vi "SWITCH Action-Status Calibrate.vi"(8 "error in (no error)":errorcluster, 10 "Message Data":variant, 11 "Data Cluster in":T1={"Tango HW"={"VISA resource"="", "Baud Rate (115200)"=2, "lAnInterfaceType"=0, "bAShowProt"=15}, "Writer Queue"=refnum, "Status"=FALSE, "Abs Position"=[], "Axis Velocity"={"dX"=0.0, "dY"=0.0, "dZ"=0.0, "dA"=0.0}, "acceleration "=0.0, "Z direction"=enum."Up", "Position Mode"="", "plLSID"=0}) -> (0 "error out":errorcluster, 3 "Data Cluster out":T1={"Tango HW"={"VISA resource"="", "Baud Rate (115200)"=2, "lAnInterfaceType"=0, "bAShowProt"=15}, "Writer Queue"=refnum, "Status"=FALSE, "Abs Position"=[], "Axis Velocity"={"dX"=0.0, "dY"=0.0, "dZ"=0.0, "dA"=0.0}, "acceleration "=0.0, "Z direction"=enum."Up", "Position Mode"="", "plLSID"=0})   [LabVIEW 2020, in "MOTOR.lvlib"]
uses:
  MOTOR.lvlib
  PS Hardware Configuration.ctl
  support/Message Queue/Message Cluster.ctl
  support/HW Message Cluster.ctl
  support/PCT FGV CMD.ctl
  support/Message Queue/Enqueue Message (Single).vi
  support/Message Queue/Message Queue.lvlib
  <instrlib>/Tango_DLL/Tango_DLL.lvlib
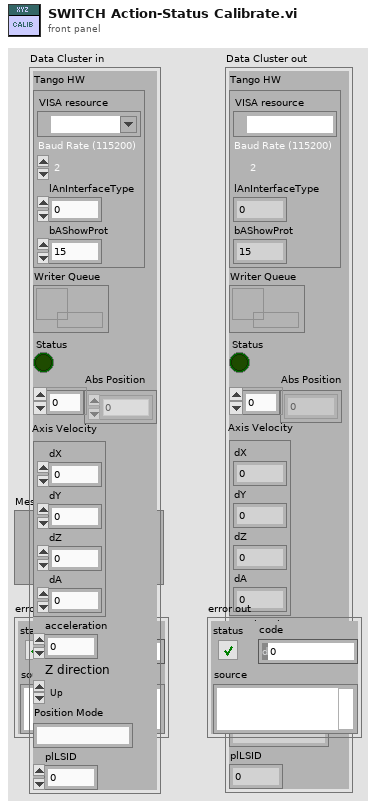
[diagram p1: front panel]
types:
  T1 = typedef "MOTOR.lvlib/PS Hardware Configuration.ctl" = cluster{"Tango HW":cluster{"VISA resource":refnum<visa-resource-name>, "Baud Rate (115200)":i32, "lAnInterfaceType":i32, "bAShowProt":i32}, "Writer Queue":refnum<queue>, "Status":bool, "Abs Position":i32[], "Axis Velocity":cluster{"dX":dbl, "dY":dbl, "dZ":dbl, "dA":dbl}, "acceleration ":dbl, "Z direction":enum16{"Up", "Down"}, "Position Mode":string, "plLSID":i32}
  T2 = typedef "PCT FGV CMD.ctl" = enum16{"INIT", "GET", "SET"}
  T3 = typedef "Message Queue.lvlib/HW Message Cluster.ctl" = cluster{"Writer Queue":refnum<queue>, "Writer Data":T4}
  T4 = typedef "Message Queue.lvlib/Message Cluster.ctl" = cluster{"Message":string, "Message Data":variant}
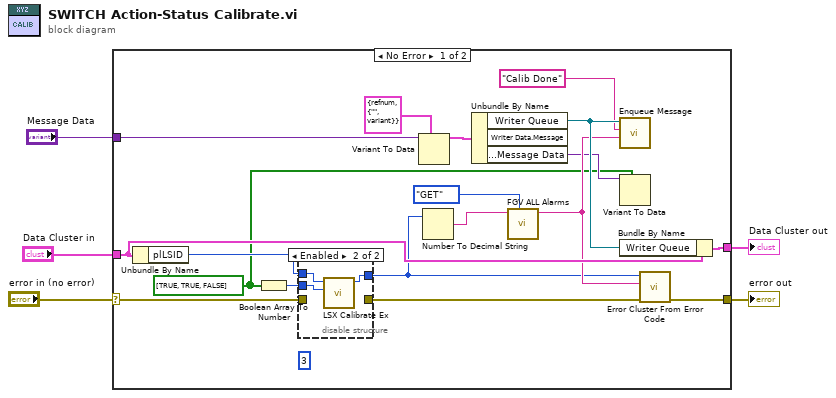
[diagram p0: block diagram]
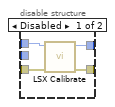
[diagram p2: hidden frame]
diagram:
  n1 = case shown="No Error" "error in (no error)" {
    selector: "error in (no error)" -> [w11 w31]
    tunnel: "Message Data" -> [w19 _]
    tunnel: [w20 w32] -> w4
    tunnel: "Data Cluster in" -> [w21 w32]
    tunnel: [w16 w31] -> w2
    frame No Error {
      (unwired) 3 ("lFlags")
      w6 = bool[] [TRUE, TRUE, FALSE]
      n2 = Unbundle By Name(w21) -> ("plLSID"=w12:i32)
      n3 = Boolean Array To Number(Boolean array=w6) -> (number=w7:u32)
      n4 = disable-structure shown="Enabled" {
        disable-tunnel: w12 -> [w27 w30]
        disable-tunnel: w11 -> [w26 _]
        disable-tunnel: [w25 w29] -> w10
        disable-tunnel: [w24 _] -> w9
        disable-tunnel: w7 -> [_ w28]
        frame Disabled {
          n5 = call <instrlib>:"LSX Calibrate.vi"("error in (no error)"=w26, "lLSID"=w27) -> ("error out"=w24:errorcluster, "function return"=w25:i32)  [unwired: 8 in]
        }
        frame Enabled {
          n6 = call <instrlib>:"LSX Calibrate Ex.vi"("lFlags"=w28, "lLSID"=w30) -> ("function return"=w29:i32)  [unwired: 8 in, 1 out]
        }
      }
      n7 = Variant To Data(type=T3 {"Writer Queue"=refnum, "Writer Data"={"Message"="", "Message Data"=variant}}, Variant=w19) -> (data=w22:T3)  [unwired: 1 in, 1 out]
      n8 = Number To Decimal String(number=w10) -> (decimal integer string=w17:string)  [unwired: 1 in]
      n9 = Unbundle By Name(w22) -> ("Writer Queue"=w15:refnum<queue>, "Writer Data.Message Data"=w8:variant)  [unwired: 1 out]
      n10 = call "FGV ALL Alarms.vi"("CMD"=PCT_FGV_CMD."GET", "name"=w17) -> ("Alarm MSG out"=w13:string)  [unwired: 8 in, 1 out]
      n11 = call-poly "Enqueue Message.vi"("Message Data"=w13, "Message"="Calib Done", "Message Queue"=w15) -> ()  [unwired: 7 in, 2 out]
      n12 = Variant To Data(type=w6, Variant=w8) -> ()  [unwired: 1 in, 2 out]
      n13 = Bundle By Name(cluster=w21, "Writer Queue"=w15) -> (w20:T1)
      n14 = call <vilib>:"Error Cluster From Error Code.vi"("error in (no error)"=w9, "error message (\"\")"=w13, "error code (0)"=w10) -> ("error out"=w16:errorcluster)  [unwired: 6 in]
    }
    frame Error {
    }
  }
  "Data Cluster out" <- w4
  "error out" <- w2
